vi "format set font size.vi"(8 "error in (no error)":errorcluster, 10 "size":dbl, 11 "format":u32) -> (0 "error out":errorcluster)   [LabVIEW 8.6]
doc: "void format_set_font_size(lxw_format format, double size);"
uses:
  pending_lvxlsxwriter/xlsxwriter.dll
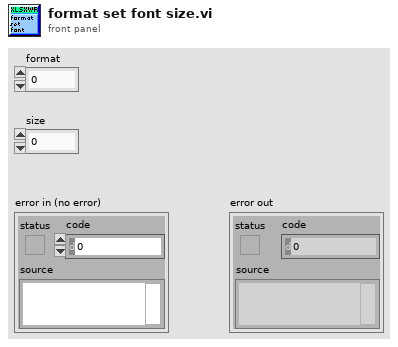
[diagram p1: front panel]
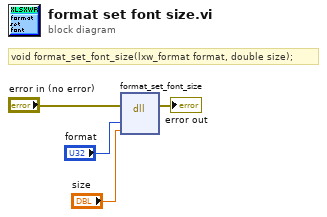
[diagram p0: block diagram]
diagram:
  # "void format_set_font_size(lxw_format format, double size);"
  n1 = dll-call lib="C:/Users/WDAGUtilityAccount/Desktop/pending_lvxlsxwriter/xlsxwriter.*" fn="format_set_font_size"(error in="error in (no error)", "format"="format", "size"="size") -> (error out=→"error out":errorcluster)  [unwired: 5 in, 1 out]
